vi "Get Configuration.vi"(8 "error in":errorcluster, 10 "Display":string(combo), 11 "VISA resource name in":refnum<visa-resource-name>) -> (0 "error out":errorcluster, 1 "Resolution":dbl, 2 "Range":dbl, 3 "VISA resource name out":refnum<visa-resource-name>, 4 "Temp":string, 5 "Function":string)   [LabVIEW 2021, in "Keysight U1282A.lvlib"]
doc: "El comando de configuración del instrumento (CONF?) regresa una serie de campos separados por commas indicando la función de medición de la pantalla principal o la secundaria. Dependiendo de la función de medición puede proporcionar la información de rango y resolución de la medición."
uses:
  Keysight U1282A.lvlib
panel:
  out "Array":string[](array[string])
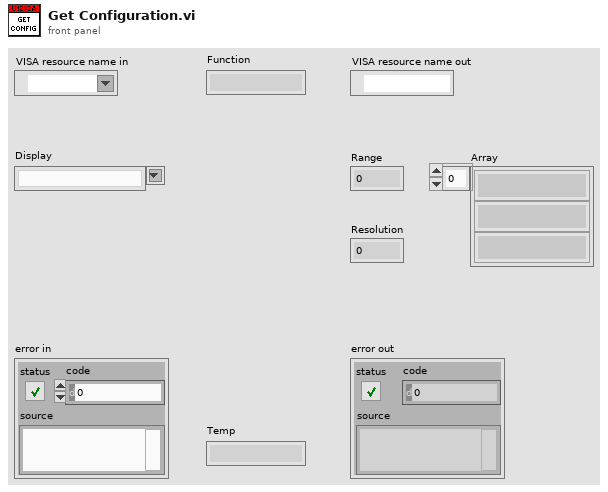
[diagram p1: front panel]
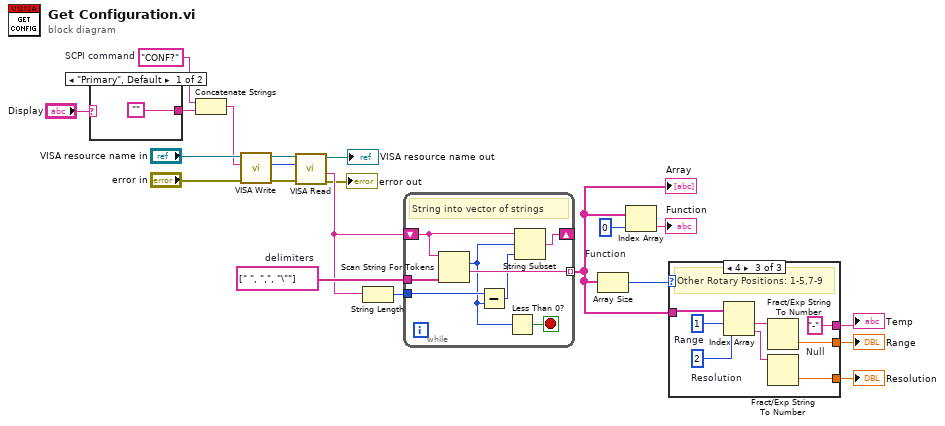
[diagram p0: block diagram]
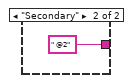
[diagram p2: hidden frame]
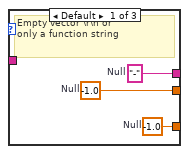
[diagram p3: hidden frame]
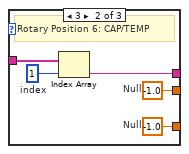
[diagram p4: hidden frame]
diagram:
  w7 = 0  # Function
  w11 = string[] [" ", ",", "\""]  # delimiters
  w14 = "CONF?"  # SCPI command
  n1 = case shown="\"Primary\", Default" "Display" {
    tunnel: ["" " @2"] -> w15
    frame "Primary", Default {
    }
    frame "Secondary" {
    }
  }
  n2 = Concatenate Strings(w14, w15) -> (w13:string)
  n3 = call "VISA Write.vi"("error in"="error in", "SCPI command"=w13, "VISA resource in"="VISA resource name in") -> ("error out"=w21:errorcluster, "Bytes at Port out"=w17:u32, "VISA resource out"=w18:refnum<visa-resource-name>)  [unwired: 6 in]
  n4 = call "VISA Read.vi"("error in"=w21, "Bytes at Port in"=w17, "VISA resource in"=w18) -> ("error out"=→"error out":errorcluster, "Reading"=w10:string, "VISA resource out"=→"VISA resource name out":refnum<visa-resource-name>)  [unwired: 5 in, 1 out]
  n5 = String Length(string=w10) -> (length=w9:i32)
  n6 = while {
    tunnel: w11 -> [w31]
    tunnel: [w30] -> w6 mode=indexing
    shift-right: [w29] -> _
    shift-left: w10 -> [w24]
    tunnel: w9 -> [w28]
    stop <- w25 stop-if-true
    # "String into vector of strings"
    n7 = Scan String For Tokens(6:w31, 9:w24) -> (1:w30:string, 2:w26:i32)  [unwired: 4 in, 2 out]
    n8 = Subtract(x=w28, y=w26) -> (x-y=w27:i32)
    n9 = Less Than 0?(x=w26) -> (x < 0?=w25:bool)
    n10 = String Subset(string=w24, offset (0)=w26, length (rest)=w27) -> (substring=w29:string)
  }
  "Array" <- w6
  n11 = Array Size(array=w6) -> (size(s)=w5:i32)
  n12 = Index Array(array=w6, index=w7) -> (element=→"Function":string)
  n13 = case shown="4" w5 {
    tunnel: w6 -> [_ w39 w47]
    tunnel: [w32 w35 w42] -> w4
    tunnel: [w33 w36 w41] -> w3
    tunnel: [w34 w37 w40] -> w2
    frame Default {
      w32 = -1.0  # Null
      w33 = -1.0  # Null
      w34 = "-"  # Null
      # "Empty vector \\r\\n or \nonly a function string"
    }
    frame 3 {
      w35 = -1.0  # Null
      w36 = -1.0  # Null
      w38 = 1  # index
      # "Rotary Position 6: CAP/TEMP"
      n14 = Index Array(array=w39, index=w38) -> (element=w37:string)
    }
    frame 4 {
      w40 = "-"  # Null
      w44 = 2  # Resolution
      w45 = 1  # Range
      # "Other Rotary Positions: 1-5,7-9"
      n15 = Index Array(array=w47, index #1=w45, index #2=w44) -> (element #1=w46:string, element #2=w43:string)
      n16 = Fract/Exp String To Number(string=w46) -> (number=w41:dbl)  [unwired: 3 in, 1 out]
      n17 = Fract/Exp String To Number(string=w43) -> (number=w42:dbl)  [unwired: 3 in, 1 out]
    }
  }
  "Range" <- w3
  "Resolution" <- w4
  "Temp" <- w2
